vi "Practica 1.vi"() -> ()   [LabVIEW 2020]
panel:
  out "Waveform Chart 2":dbl[](graph)
  out "Frecuencia":dbl format="%#_13g"
  out "Waveform Chart":dynamicdata(graph)
  in  "stop":bool
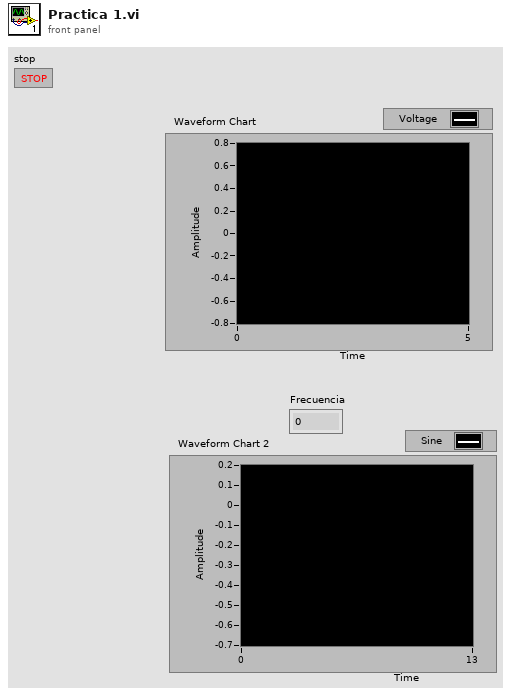
[diagram p1: front panel]
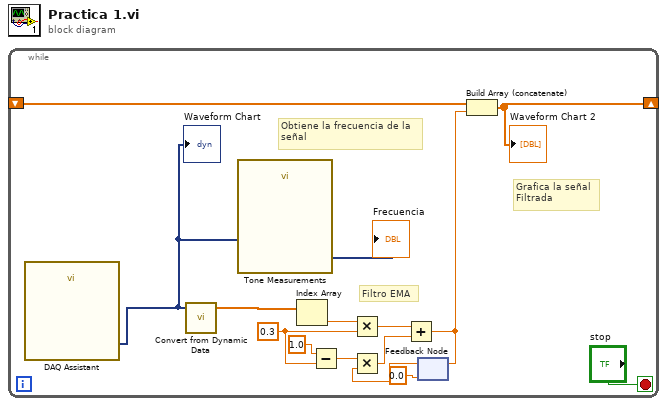
[diagram p0: block diagram]
diagram:
  n1 = while {
    shift-right: [w2] -> _
    shift-left: _ -> [w3]
    stop <- "stop" stop-if-true
    w13 = 0.3 ("y")
    # "Grafica la señal \nFiltrada"
    # "Filtro EMA"
    # "Obtiene la frecuencia de la\nseñal"
    n2 = call "DAQ Assistant"() -> ("data"=w1:dynamicdata)  [unwired: 16 in, 3 out]
    "Waveform Chart" <- w1
    n3 = call "Convert from Dynamic Data"("Dynamic Data Type"=w1) -> ("Array"=w6:dbl[])  [unwired: 3 in]
    n4 = call "Tone Measurements"("Signals"=w1) -> ("Frequency"=→"Frecuencia":dynamicdata)  [unwired: 9 in, 1 out]
    n5 = Index Array(array=w6) -> (element=w5:dbl)  [unwired: 1 in]
    n6 = Subtract(x=1.0, y=w13) -> (x-y=w11:dbl)
    n7 = Multiply(x=w5, y=w13) -> (x*y=w9:dbl)
    n8 = feedback #1(0.0) -> (w8:dbl)
    n9 = Multiply(x=w11, y=w8) -> (x*y=w10:dbl)
    n10 = Add(x=w9, y=w10) -> (x+y=w4:dbl)
    n11 = feedback-in #1(w4) -> ()
    n12 = Build Array (concatenate)(w3, w4) -> (w2:dbl[])
    "Waveform Chart 2" <- w2
  }
